vi "Valve_Position.vi"(0 "Data in":T1, 2 "NewVal":dbl, 3 "error in":errorcluster) -> (5 "Data out":T1, 6 "State":T2, 7 "error out":errorcluster)   [LabVIEW 2023]
uses:
  Controls/DataCluster.ctl
  Controls/State.ctl
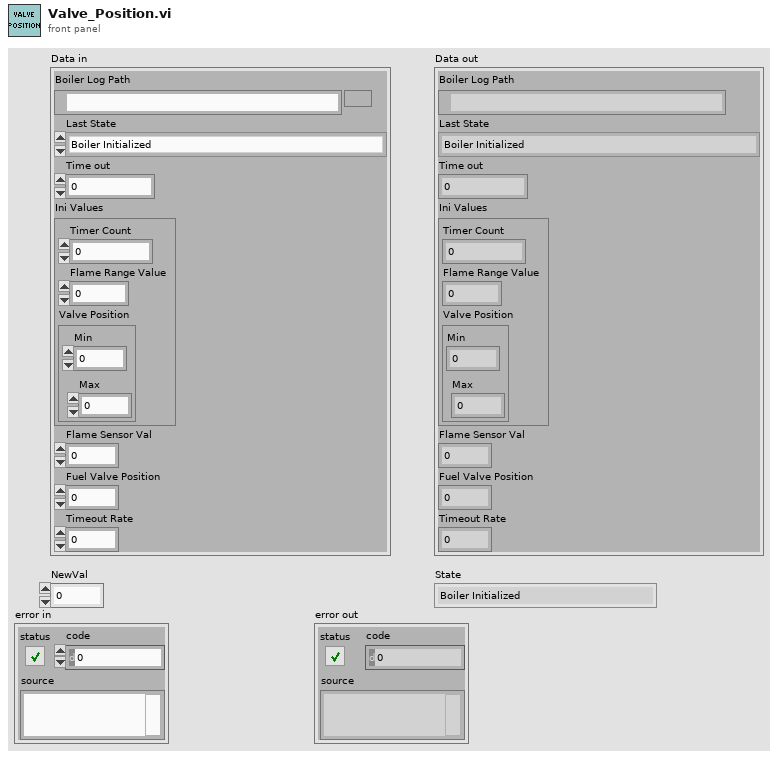
[diagram p1: front panel]
types:
  T1 = typedef "DataCluster.ctl" = cluster{"Boiler Log Path":path, "Last State":T2, "Time out":i32, "Ini Values":cluster{"Timer Count":dbl, "Flame Range Value":dbl, "Valve Position ":cluster{"Min":dbl, "Max":dbl}}, "Flame Sensor Val":dbl, "Fuel Valve Position":dbl, "Timeout Rate":i32}
  T2 = typedef "State.ctl" = enum16{"Boiler Initialized", "Boiler Ready", "Start Pre-Purge", "Pre-Purge Complete", "Pilot On", "Pilot Proved", "Force Draft Fan ON", "Boiler Running", "Start Shutdown Purge", "Shutdown Purge Complete", "Wait for Something"}
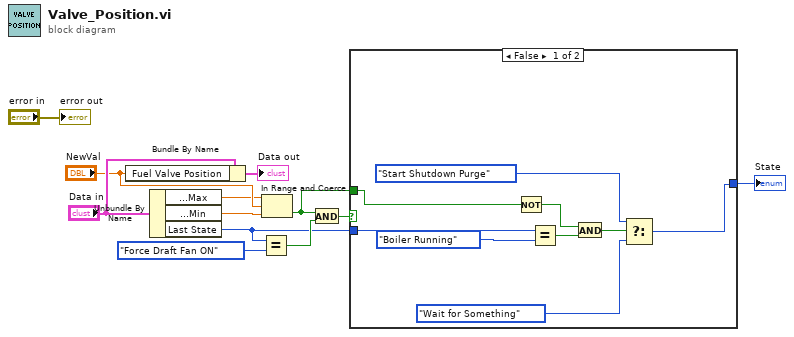
[diagram p0: block diagram]
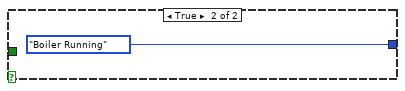
[diagram p2: hidden frame]
diagram:
  n1 = Bundle By Name(cluster="Data in", "Fuel Valve Position"="NewVal") -> (→"Data out":T1)
  n2 = Unbundle By Name("Data in") -> ("Ini Values.Valve Position.Max"=w8:dbl, "Ini Values.Valve Position.Min"=w9:dbl, "Last State"=w2:T2)
  n3 = Equal?(x=w2, y=State."Force Draft Fan ON") -> (x = y?=w5:bool)
  n4 = In Range and Coerce(upper limit=w8, x="NewVal", lower limit=w9) -> (In Range?=w1:bool)  [unwired: 1 out]
  n5 = And(x=w1, y=w5) -> (x .and. y?=w4:bool)
  n6 = case shown="False" w4 {
    tunnel: [w14 State."Boiler Running"] -> w3
    tunnel: w2 -> [w21 _]
    tunnel: w1 -> [w18 _]
    frame False {
      n7 = Not(x=w18) -> (.not. x?=w17:bool)
      n8 = Equal?(x=w21, y=State."Boiler Running") -> (x = y?=w19:bool)
      n9 = And(x=w17, y=w19) -> (x .and. y?=w16:bool)
      n10 = Select(t=State."Start Shutdown Purge", s=w16, f=State."Wait for Something") -> (s? t:f=w14:T2)
    }
    frame True {
    }
  }
  "State" <- w3
  "error out" <- "error in"
